vi "Populating the Asynchronous Call and Collect Pool.vi"() -> ()   [LabVIEW 2020]
doc: "<b>Example Description</b>\n\nThis example shows the difference in performance between pre-populating the asynchronous call pool or not. Pre-populating the pool will prevent the Start Asynchronous Call node from needing to switch to the LabVIEW UI thread and create a data space.\n\nWhen running this example, you can see the time it takes to start asynchronous calls is less when the asynchronous call pool was properly pre-populated.\n\n<b>Overview of Asynchronous Call Pool</b>\n\nWhen performing asynchronous calls, an asynchronous call pool of data spaces is automatically created by the Open VI Reference function. By default, the call pool will be sized based on the number of computer cores.\n\nWhen the Start Asynchronous Call node is called, it will attempt to retrieve a data space from the asynchronous call pool. If there are no data spaces available, the Start Asynchronous Call node will automatically create a data space on demand and add it to the pool. This data space creation must be done in the LabVIEW UI thread. The Start Asynchronous Call node will only require the UI thread when it needs to create a data space.\n\nData spaces are automatically returned to the asynchronous call pool differently depending on whether you are performing a call and collect or a call and forget. For the call and collect use case, this is done only after the Wait On Asynchronous Call completes and results have been collected. For the call and forget use case, this is done as soon as the target VI execution completes.\n\nBecause the Start Asynchronous call node can add data spaces to the pool on demand, this can cause short delays when starting a call. These delays can be avoided by using the Populate Asynchronous Call Pool method to create data spaces beforehand."
panel:
  out "error out":errorcluster
  in  "milliseconds to wait":u32
  out "Current Size":i32
  out "Asynch index":i32[](array[numeric])
  out "sorted x + y":dbl[](array[numeric])
  out "sorted asynch x + y":dbl[](array[numeric])
  out "sorted x = y?":bool
  out "x = y?":bool
  out "Numeric 2":i32
  out "Numeric":i32
  out "x+y":dbl[](array[numeric])
  out "Asynch x+ y":dbl[](array[numeric])
  in  "Number of calls":i32=100
  out "Preallocate Pool -- Time to start all calls (ms)":u32
  # "Overview: Demonstrates the use of the  Populate Asynchronous Call Pool method with Asynchronous VI Call AND COLLECT.\nInstructions:\nRun the VI. Observe the benchmark values below. See the block diagram for more information."
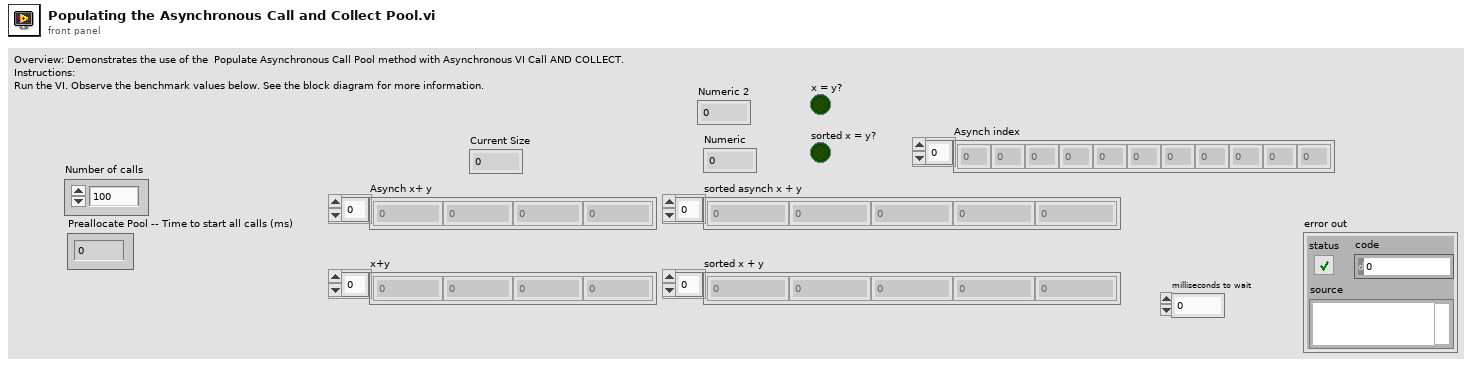
[diagram p1: front panel]
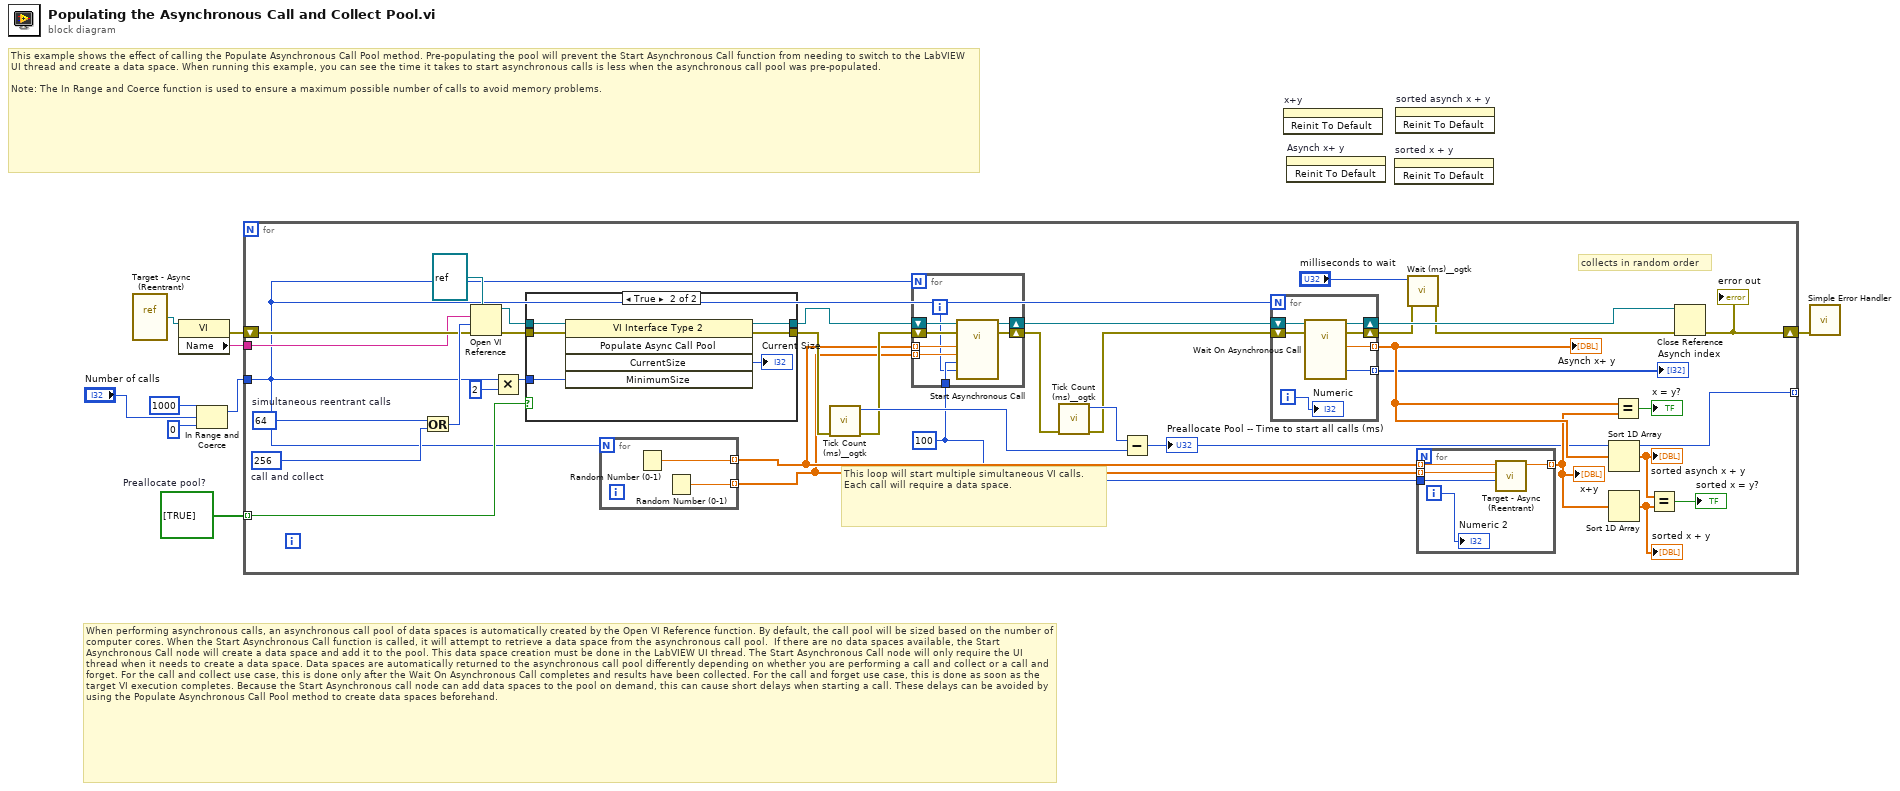
[diagram p0: block diagram]
diagram:
  w9 = bool[] [TRUE]  # Preallocate pool?
  # "When performing asynchronous calls, an asynchronous call pool of data spaces is automatically created by the Open VI Reference function. By default, the call pool will be sized based on the number of computer cores. When the Start Asynchronous Call function is called, it will attempt to retrieve a data space from the asynchronous call pool.  If there are no data spaces available, the Start Asynchronous Call node will create a data space and add it to the pool. This data space creation must be done in the LabVIEW UI thread. The Start Asynchronous Call node will only require the UI thread when it needs to create a data space. Data spaces are automatically returned to the asynchronous call pool differently depending on whether you are performing a call and collect or a call and forget. For the call and collect use case, this is done only after the Wait On Asynchronous Call completes and results have been collected. For the call and forget use case, this is done as soon as the target VI execution completes. Because the Start Asynchronous call node can add data spaces to the pool on demand, this can cause short delays when starting a call. These delays can be avoided by using the Populate Asynchronous Call Pool method to create data spaces beforehand."
  # "This example shows the effect of calling the Populate Asynchronous Call Pool method. Pre-populating the pool will prevent the Start Asynchronous Call function from needing to switch to the LabVIEW UI thread and create a data space. When running this example, you can see the time it takes to start asynchronous calls is less when the asynchronous call pool was pre-populated.\n\nNote: The In Range and Coerce function is used to ensure a maximum possible number of calls to avoid memory problems."
  n1 = vi-ref "Target - Async (Reentrant).vi"() -> (w3:refnum<vi>)
  n2 = property class="VI"(reference=w3) -> (error out=w2:errorcluster, "Name"=w1:string)  [unwired: 1 in, 1 out]
  n3 = In Range and Coerce(upper limit=1000 ("y"), x="Number of calls", lower limit=0) -> (coerced(x)=w5:i32)  [unwired: 1 out]
  n4 = for {
    tunnel: [w17] -> _ mode=indexing
    tunnel: w9 -> [w38] mode=indexing
    tunnel: w5 -> [w10]
    shift-right: [w44] -> w4
    shift-left: w2 -> [w36]
    tunnel: w1 -> [w35]
    w24 = u32 100 ("Wait (Milliseconds)")
    w37 = 64  # simultaneous reentrant calls
    w43 = 256  # call and collect
    # "collects in random order"
    # "This loop will start multiple simultaneous VI calls. Each call will require a data space."
    n5 = Or(x=w37, y=w43) -> (x .or. y?=w42:i32)
    n6 = Open VI Reference(type specifier VI Refnum (for type only)=refnum<vi> refnum, vi path=w35, options=w42, error in (no error)=w36) -> (vi reference=w41:refnum<vi>, error out=w40:errorcluster)  [unwired: 2 in]
    n7 = Multiply(x=w10, y=2) -> (x*y=w15:i32)
    n8 = case shown="True" w38 {
      tunnel: w41 -> [w69 w75]
      tunnel: w40 -> [w68 w74]
      tunnel: [w69 w73] -> w39
      tunnel: [w68 w72] -> w33
      tunnel: w15 -> [_ w71]
      frame False {
      }
      frame True {
        n9 = invoke class="VI Interface Type 2" method="Populate Async Call Pool"(reference=w75, error in=w74, "MinimumSize"=w71) -> (reference out=w73:refnum<vi>, error out=w72:errorcluster, "CurrentSize"=→"Current Size":i32)  [unwired: 2 in, 2 out]
      }
    }
    n10 = for {
      N: w10 -> [_]
      tunnel: [w52] -> w26 mode=indexing
      tunnel: [w51] -> w25 mode=indexing
      n11 = Random Number (0-1)() -> (number: 0 to 1=w52:dbl)
      n12 = Random Number (0-1)() -> (number: 0 to 1=w51:dbl)
    }
    n13 = call <userlib>:"Tick Count (ms)__ogtk.vi"("error in (no error)"=w33) -> ("error out"=w31:errorcluster, "millisecond timer value"=w32:u32)  [unwired: 9 in]
    n14 = for {
      N: w10 -> [_]
      shift-right: [w60] -> w30
      shift-left: w31 -> [w57]
      shift-right: [w59] -> w34
      shift-left: w39 -> [w58]
      tunnel: w26 -> [w56] mode=indexing
      tunnel: w25 -> [w55] mode=indexing
      tunnel: w24 -> [w54]
      i -> [w53]
      n15 = call-by-ref "Start Asynchronous Call"(reference=w58, error in=w57, "index"=w53, "Wait (Milliseconds)"=w54, "Y"=w55, "X"=w56) -> (reference out=w59:refnum<vi>, error out=w60:errorcluster)  [unwired: 6 in, 2 out]
    }
    n16 = call <userlib>:"Tick Count (ms)__ogtk.vi"("error in (no error)"=w30) -> ("error out"=w28:errorcluster, "millisecond timer value"=w29:u32)  [unwired: 9 in]
    n17 = Subtract(x=w29, y=w32) -> (x-y=w17:u32)
    "Preallocate Pool -- Time to start all calls (ms)" <- w17
    n18 = for {
      N: w10 -> [_]
      shift-right: [w64] -> w13
      shift-left: w28 -> [w66]
      shift-right: [w65] -> w27
      shift-left: w34 -> [w67]
      tunnel: [w63] -> w22 mode=indexing
      tunnel: [w61] -> w16 mode=indexing
      i -> [w62]
      n19 = call-by-ref "Wait On Asynchronous Call"(reference=w67, error in=w66) -> (reference out=w65:refnum<vi>, error out=w64:errorcluster, "index out"=w61:i32, "X + Y"=w63:dbl)  [unwired: 10 in]
      "Numeric" <- w62
    }
    "Asynch x+ y" <- w22
    "Asynch index" <- w16
    n20 = call <userlib>:"Wait (ms)__ogtk.vi"("error in (no error)"=w13, "milliseconds to wait"="milliseconds to wait") -> ("error out"=w12:errorcluster)  [unwired: 8 in, 1 out]
    n21 = for {
      tunnel: w26 -> [w50] mode=indexing
      tunnel: w25 -> [w49] mode=indexing
      tunnel: w24 -> [w48]
      tunnel: [w47] -> w21 mode=indexing
      i -> [w46]
      n22 = call "Target - Async (Reentrant).vi"("Wait (Milliseconds)"=w48, "Y"=w49, "X"=w50) -> ("X + Y"=w47:dbl)  [unwired: 7 in, 1 out]
      "Numeric 2" <- w46
    }
    "x+y" <- w21
    n23 = Sort 1D Array(array=w22) -> (sorted array=w19:dbl[])
    "sorted asynch x + y" <- w19
    n24 = Sort 1D Array(array=w21) -> (sorted array=w20:dbl[])
    "sorted x + y" <- w20
    n25 = Equal?(x=w22, y=w21) -> (x = y?=→"x = y?":bool)
    n26 = Equal?(x=w19, y=w20) -> (x = y?=→"sorted x = y?":bool)
    n27 = Close Reference(reference=w27, error in (no error)=w12) -> (error out=w44:errorcluster)
    "error out" <- w44
  }
  n28 = invoke on="x+y" class="Arr (strict)" method="Reinit To Default"() -> ()  [unwired: 3 in, 3 out]
  n29 = invoke on="Asynch x+ y" class="Arr (strict)" method="Reinit To Default"() -> ()  [unwired: 3 in, 3 out]
  n30 = invoke on="sorted x + y" class="Arr (strict)" method="Reinit To Default"() -> ()  [unwired: 3 in, 3 out]
  n31 = invoke on="sorted asynch x + y" class="Arr (strict)" method="Reinit To Default"() -> ()  [unwired: 3 in, 3 out]
  n32 = call <vilib>:"Simple Error Handler.vi"("error in (no error)"=w4) -> ()  [unwired: 4 in, 5 out]
